vi "Request Pref State.vi"(8 "error in (no error)":errorcluster, 11 "PluginGUI in":refnum<class "PluginGUI.lvclass">) -> (0 "error out":errorcluster, 3 "PluginGUI out":refnum<class "PluginGUI.lvclass">)   [LabVIEW 2020, in "VolatusGUI.lvlib" / "PluginGUI.lvclass"]
uses:
  PluginGUI.lvclass
  C:/dev/lv20CE/relink/lv-volatus/Volatus/Module/Module.lvclass
  GUI Manager Identity/GUI Manager Identity.lvclass
  C:/dev/lv20CE/relink/lv-volatus/Volatus/Identity/Identity.lvclass
  Volatus/Module/Module.lvclass/Module.ctl
  GUIStateValue/GUIStateValue.lvclass
  C:/dev/lv20CE/relink/lv-promises/Promises/Value/Value.lvclass
  PluginGUI.lvclass/PluginGUI.ctl
  Volatus/MessageQ/MessageQ.lvclass/MessageQ.ctl
  Volatus/Module/Self Q.vi
  Volatus/MessageQ/Send.vi
  Volatus/VolatusAPI/VolatusAPI.lvclass
  Volatus/Module/Module.lvclass
  Volatus/MessageQ/MessageQ.lvclass
  C:/dev/lv20CE/relink/lv-volatus/VolatusGUI/PluginGUI/PluginGUI.lvclass
  C:/dev/lv20CE/relink/lv-volatus/VolatusGUI/GUIStateValue/GUIStateValue.lvclass
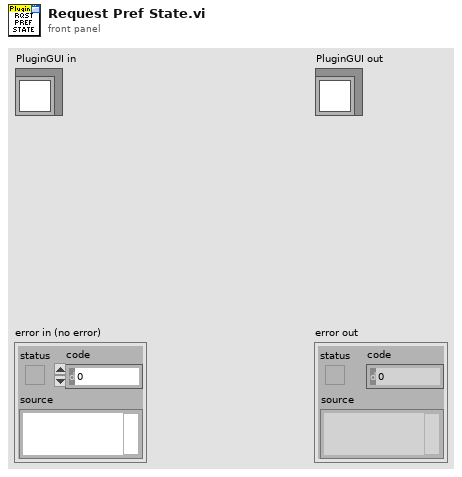
[diagram p1: front panel]
types:
  T1 = typedef "VolatusGUI.lvlib/GUI State.ctl" = cluster{"GUI ID":string, "Visible":bool, "Visibility Set":bool, "Bounds":T2, "Bounds Set":bool}
  T2 = typedef "LVRectTypeDef.ctl" = cluster{"Left":i16, "Top":i16, "Right":i16, "Bottom":i16}
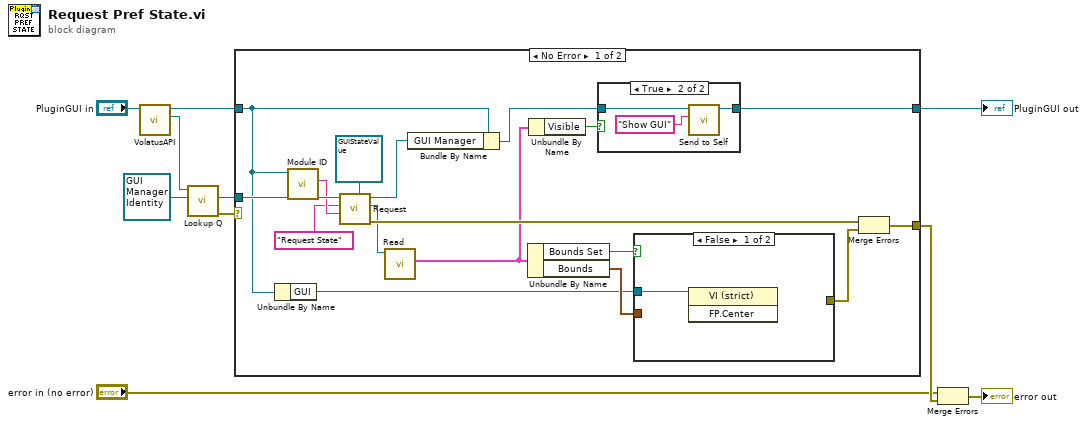
[diagram p0: block diagram]
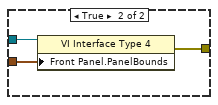
[diagram p2: hidden frame]
diagram:
  n1 = call "VolatusAPI.vi"("Module in"="PluginGUI in") -> ("VolatusAPI"=w9:refnum<class "VolatusAPI.lvclass">, "Module out"=w7:refnum<class "PluginGUI.lvclass">)  [unwired: 9 in]
  n2 = call "Lookup Q.vi"("Identity"=refnum<class "GUI Manager Identity.lvclass"> refnum ("VolatusGUI:GUI Manager Identity.lvclass"), "VolatusAPI in"=w9) -> ("error out"=w6:errorcluster, "MessageQ"=w5:refnum<class "MessageQ.lvclass">)  [unwired: 7 in, 1 out]
  n3 = case shown="No Error" w6 {
    tunnel: w7 -> [w12 w36]
    tunnel: w5 -> [w26 _]
    tunnel: [w14 w36] -> w4
    tunnel: [w13 _] -> w3
    frame No Error {
      n4 = Unbundle By Name(w12) -> ("GUI"=w11:refnum<vi>)
      n5 = call-dynamic "Module ID.vi"("Module in"=w12) -> ("Module ID"=w25:string)  [unwired: 10 in]
      n6 = call "Request.vi"("Response Value Type"=refnum<class "GUIStateValue.lvclass"> refnum ("VolatusGUI:GUIStateValue.lvclass"), "Data"=w25, "ID"="Request State", "MessageQ in"=w26) -> ("error out"=w27:errorcluster, "Response"=w22:refnum<class "GUIStateValue.lvclass">, "MessageQ out"=w19:refnum<class "MessageQ.lvclass">)  [unwired: 5 in]
      n7 = call "Read.vi"("GUIStateValue in"=w22) -> ("GUI State"=w18:T1)  [unwired: 10 in]
      n8 = Bundle By Name(cluster=w12, "GUI Manager"=w19) -> (w20:refnum<class "PluginGUI.lvclass">)
      n9 = Unbundle By Name(w18) -> ("Bounds Set"=w17:bool, "Bounds"=w16:T2)
      n10 = Unbundle By Name(w18) -> ("Visible"=w21:bool)
      n11 = case shown="True" w21 {
        tunnel: w20 -> [w32 w35]
        tunnel: [w32 w33] -> w14
        frame False {
        }
        frame True {
          n12 = call "Send to Self.vi"("Message ID"="Show GUI", "Module in"=w35) -> ("Module out"=w33:refnum<class "PluginGUI.lvclass">)  [unwired: 8 in, 1 out]
        }
      }
      n13 = case shown="False" w17 {
        tunnel: w11 -> [w28 w31]
        tunnel: w16 -> [_ w30]
        tunnel: [_ w29] -> w15
        frame False {
          n14 = invoke class="VI (strict)" method="FP.Center"(reference=w28) -> ()  [unwired: 2 in, 3 out]
        }
        frame True {
          n15 = property class="VI Interface Type 4"(reference=w31, "Front Panel.PanelBounds"=w30) -> (error out=w29:errorcluster)  [unwired: 1 in, 1 out]
        }
      }
      n16 = Merge Errors(w27, w15) -> (w13:errorcluster)
    }
    frame Error {
      # "GUI Manager not running, don't worry about pref state"
    }
  }
  "PluginGUI out" <- w4
  n17 = Merge Errors("error in (no error)", w3) -> (→"error out":errorcluster)
